vi "Test_IMU.vi"() -> ()   [LabVIEW 2014]
uses:
  <userlib>/UCSD Robotics Lab/Robotics-Cape/LV/libroboticscape.lvlib
panel:
  out "Timing Block":T1 {"Actual Hz" format="%#_3g"; "Dt" format="%#_4g"; "Average Hz" format="%#_4g"}
  out "Gyro (Mode/sec)":T2 {"gyro[0]" format="%#_3g"; "gyro[1]" format="%#_3g"; "gyro[2]" format="%#_3g"}
  out "Accel (m/s^2)":T3 {"accel[0]" format="%#_3g"; "accel[1]" format="%#_3g"; "accel[2]" format="%#_3g"}
  out "Temp (C)":sgl format="%#_3g"
  in  "Temp On/Off":bool
  in  "Mag On/Off":bool
  out "Mag Field (uT)":T4 {"mag[0]" format="%#_3g"; "mag[1]" format="%#_3g"; "mag[2]" format="%#_3g"}
  in  "Gyro On/Off":bool
  in  "Accel On/Off":bool
  in  "Mode":enum16{"Rad", "Deg", "Raw"}(ring)=enum."Deg"
  out "State":T5(ring)
  in  "stop":bool
  # "Always stop the VI using the rectangular STOP button above, never with the round stopsign (Abort)"
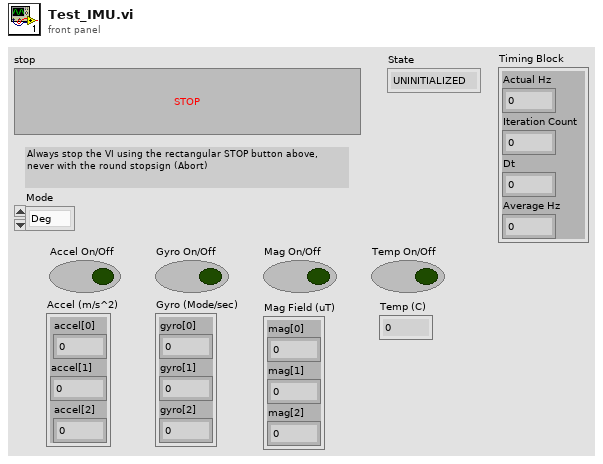
[diagram p1: front panel]
types:
  T1 = cluster{"Actual Hz":dbl, "Iteration Count":dbl, "Dt":dbl, "Average Hz":dbl}
  T2 = cluster{"gyro[0]":dbl, "gyro[1]":dbl, "gyro[2]":dbl}
  T3 = cluster{"accel[0]":sgl, "accel[1]":sgl, "accel[2]":sgl}
  T4 = cluster{"mag[0]":sgl, "mag[1]":sgl, "mag[2]":sgl}
  T5 = enum16{"UNINITIALIZED", "RUNNING", "PAUSED", "EXITING"}
  T6 = cluster{"accel[0]":sgl, "accel[1]":sgl, "accel[2]":sgl, "gyro[0]":sgl, "gyro[1]":sgl, "gyro[2]":sgl, "mag[0]":sgl, "mag[1]":sgl, "mag[2]":sgl, "temp":sgl, "raw_gyro[0]":i16, "raw_gyro[1]":i16, "raw_gyro[2]":i16, "raw_accel[0]":i16, "raw_accel[1]":i16, "raw_accel[2]":i16, "accel_to_ms2":sgl, "gyro_to_degs":sgl, "dmp_quat[0]":sgl, "dmp_quat[1]":sgl, "dmp_quat[2]":sgl, "dmp_quat[3]":sgl, "dmp_TaitBryan[0]":sgl, "dmp_TaitBryan[1]":sgl, "dmp_TaitBryan[2]":sgl, "fused_quat[0]":sgl, "fused_quat[1]":sgl, "fused_quat[2]":sgl, "fused_quat[3]":sgl, "fused_TaitBryan[0]":sgl, "fused_TaitBryan[1]":sgl, "fused_TaitBryan[2]":sgl, "compass_heading":sgl, "compass_heading_raw":sgl}
  T7 = enum16{"UNINITIALIZED", "RUNING", "PAUSED", "EXITING"}
  T8 = cluster{"raw_accel[0]":i16, "raw_accel[1]":i16, "raw_accel[2]":i16}
  T9 = cluster{"gyro[0]":sgl, "gyro[1]":sgl, "gyro[2]":sgl}
  T10 = cluster{"raw_gyro[0]":i16, "raw_gyro[1]":i16, "raw_gyro[2]":i16}
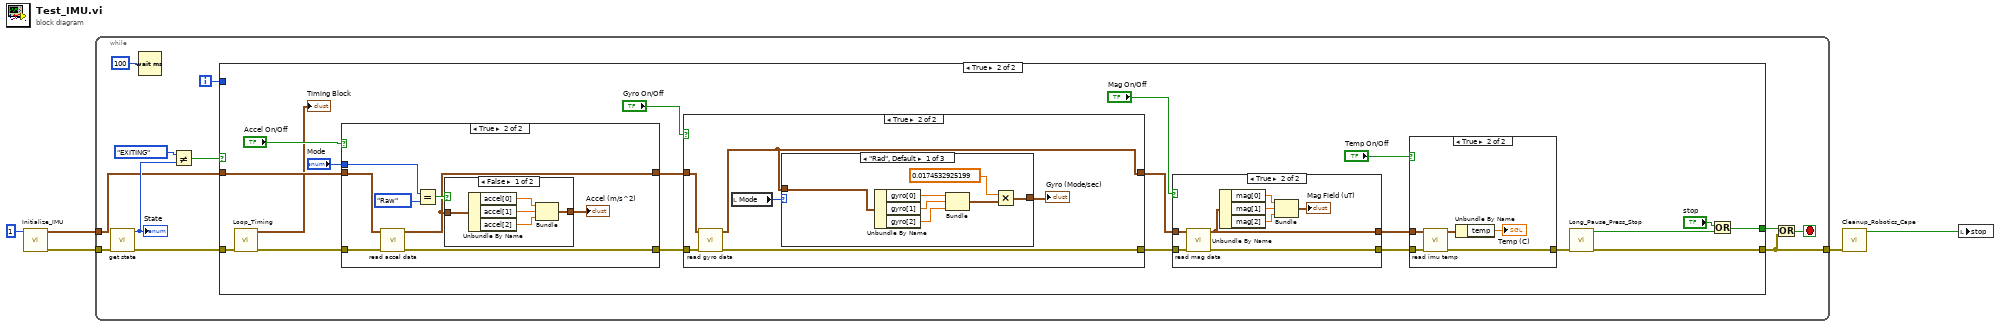
[diagram p0: block diagram]
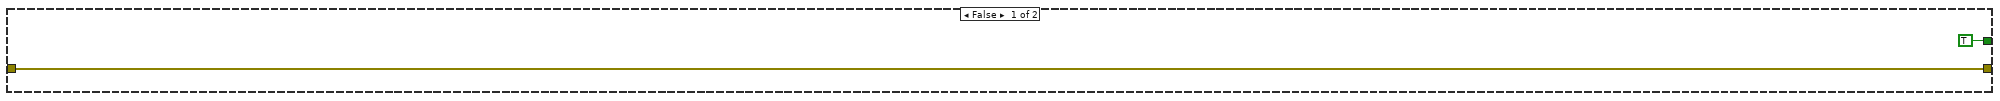
[diagram p2: hidden frame]
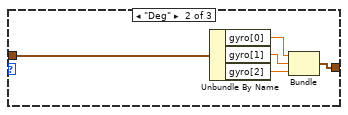
[diagram p6: hidden frame]
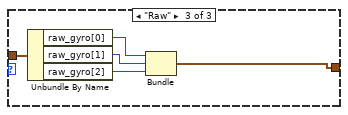
[diagram p7: hidden frame]
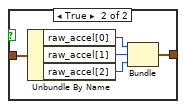
[diagram p9: hidden frame]
diagram:
  n1 = call "Initialize_IMU.vi"("enable_magnetometer"=1) -> ("error out"=w3:errorcluster, "data out"=w4:T6)  [unwired: 8 in, 1 out]
  n2 = while {
    tunnel: w3 -> [w15]
    tunnel: [w9] -> w1
    tunnel: w4 -> [w6]
    i -> [w14]
    stop <- w16 stop-if-true
    n3 = call <userlib>:"get state.vi"("error in (no error)"=w15) -> ("error out"=w10:errorcluster, "function return"=w12:u32)  [unwired: 9 in]
    "State" <- w12
    n4 = Wait (ms)(milliseconds to wait=u32 100) -> ()  [unwired: 1 out]
    n5 = Not Equal?(x=T7."EXITING" ("State 2"), y=w12) -> (x != y?=w11:bool)
    n6 = case shown="True" w11 {
      tunnel: w14 -> [_ _]
      tunnel: w10 -> [w18 w26]
      tunnel: [w18 w20] -> w9
      tunnel: [TRUE ("stop") w22] -> w8
      tunnel: w6 -> [_ w36]
      frame False {
      }
      frame True {
        n7 = call "Loop_Timing.vi"("error in"=w26) -> ("error out"=w25:errorcluster, "Timing Block"=→"Timing Block":T1)  [unwired: 9 in]
        n8 = case shown="True" "Accel On/Off" {
          tunnel: "Mode" -> [_ w89]
          tunnel: w25 -> [w81 w87]
          tunnel: w36 -> [w80 w86]
          tunnel: [w81 w84] -> w35
          tunnel: [w80 w83] -> w32
          frame False {
          }
          frame True {
            n9 = call <userlib>:"read accel data.vi"("error in (no error)"=w87, "data"=w86) -> ("error out"=w84:errorcluster, "data out"=w83:T6)  [unwired: 7 in, 1 out]
            n10 = Equal?(x=w89, y=enum16{"Rad", "Deg", "Raw"}."Raw" ("Mode")) -> (x = y?=w85:bool)
            n11 = case shown="False" w85 {
              tunnel: w83 -> [w94 w99]
              tunnel: [w90 w95] -> w82
              frame False {
                n12 = Unbundle By Name(w94) -> ("accel[0]"=w92:sgl, "accel[1]"=w93:sgl, "accel[2]"=w91:sgl)
                n13 = Bundle("accel[0]"=w92, "accel[1]"=w93, "accel[2]"=w91) -> (w90:T3)  [unwired: 1 in]
              }
              frame True {
                n14 = Unbundle By Name(w99) -> ("raw_accel[0]"=w98:i16, "raw_accel[1]"=w97:i16, "raw_accel[2]"=w96:i16)
                n15 = Bundle("raw_accel[0]"=w98, "raw_accel[1]"=w97, "raw_accel[2]"=w96) -> (w95:T8)  [unwired: 1 in]
              }
            }
            "Accel (m/s^2)" <- w82
          }
        }
        n16 = case shown="True" "Gyro On/Off" {
          tunnel: w35 -> [w56 w62]
          tunnel: w32 -> [w55 w61]
          tunnel: [w56 w60] -> w31
          tunnel: [w55 w58] -> w30
          frame False {
          }
          frame True {
            n17 = call <userlib>:"read gyro data.vi"("error in (no error)"=w62, "data"=w61) -> ("error out"=w60:errorcluster, "data out"=w58:T6)  [unwired: 7 in, 1 out]
            n18 = local read "Mode"() -> (w59:enum16{"Rad", "Deg", "Raw"})
            n19 = case shown="\"Rad\", Default" w59 {
              tunnel: w58 -> [w69 w74 w79]
              tunnel: [w64 w70 w75] -> w57
              frame "Rad", Default {
                n20 = Unbundle By Name(w69) -> ("gyro[0]"=w66:sgl, "gyro[1]"=w68:sgl, "gyro[2]"=w67:sgl)
                n21 = Bundle("gyro[0]"=w66, "gyro[1]"=w68, "gyro[2]"=w67) -> (w65:T9)  [unwired: 1 in]
                n22 = Multiply(x=0.0174532925199, y=w65) -> (x*y=w64:T2)
              }
              frame "Deg" {
                n23 = Unbundle By Name(w74) -> ("gyro[0]"=w71:sgl, "gyro[1]"=w73:sgl, "gyro[2]"=w72:sgl)
                n24 = Bundle("gyro[0]"=w71, "gyro[1]"=w73, "gyro[2]"=w72) -> (w70:T9)  [unwired: 1 in]
              }
              frame "Raw" {
                n25 = Unbundle By Name(w79) -> ("raw_gyro[0]"=w78:i16, "raw_gyro[1]"=w77:i16, "raw_gyro[2]"=w76:i16)
                n26 = Bundle("raw_gyro[0]"=w78, "raw_gyro[1]"=w77, "raw_gyro[2]"=w76) -> (w75:T10)  [unwired: 1 in]
              }
            }
            "Gyro (Mode/sec)" <- w57
          }
        }
        n27 = case shown="True" "Mag On/Off" {
          tunnel: [w46 w54] -> w38
          tunnel: w31 -> [w46 w53]
          tunnel: w30 -> [w45 w52]
          tunnel: [w45 w47] -> w28
          frame False {
          }
          frame True {
            n28 = call <userlib>:"read mag data.vi"("error in (no error)"=w53, "data"=w52) -> ("error out"=w54:errorcluster, "data out"=w47:T6)  [unwired: 7 in, 1 out]
            n29 = Unbundle By Name(w47) -> ("mag[0]"=w50:sgl, "mag[1]"=w51:sgl, "mag[2]"=w49:sgl)
            n30 = Bundle("mag[0]"=w50, "mag[1]"=w51, "mag[2]"=w49) -> (→"Mag Field (uT)":T4)  [unwired: 1 in]
          }
        }
        n31 = case shown="True" "Temp On/Off" {
          tunnel: w38 -> [w39 w44]
          tunnel: [w39 w43] -> w19
          tunnel: w28 -> [_ w42]
          frame False {
          }
          frame True {
            n32 = call <userlib>:"read imu temp.vi"("error in (no error)"=w44, "data"=w42) -> ("error out"=w43:errorcluster, "data out"=w41:T6)  [unwired: 7 in, 1 out]
            n33 = Unbundle By Name(w41) -> ("temp"=→"Temp (C)":sgl)
          }
        }
        n34 = call "Long_Pause_Press_Stop.vi"("error in (no error)"=w19) -> ("error out"=w20:errorcluster, "Stop"=w21:bool)  [unwired: 9 in]
        n35 = Or(x="stop", y=w21) -> (x .or. y?=w22:bool)
      }
    }
    n36 = Or(x=w8, y=w9) -> (x .or. y?=w16:bool)
  }
  n37 = call "Cleanup_Robotics_Cape.vi"("error in (no error)"=w1) -> ("Stop Local Variabl"=w5:bool)  [unwired: 9 in, 1 out]
  n38 = local write "stop"(w5) -> ()
